vi "dfd_Create Filter Bank Response Distortion.vi"(7 "# freq bins (512)":i32=512, 8 "error in (no error)":errorcluster, 10 "synthesis subband filtes":T1[](array[typedef]) {"mMRate_SumWl" min=1 max=32 step=1; "mMRate_InputIwl" min=1 max=32 step=1; "mMRate_GainWl" min=1 max=32 step=1; "mMRate_OutputWl" min=1 max=32 step=1; "mMRate_InputWl" min=1 max=32 step=1; "mMRate_CoefWl" min=1 max=32 step=1; "mMRate_Mode" items=["Default"=-1, "No Rate Change"=0, "Interpolation"=1, "Decimation"=2, "Interpolated"=3, "Rational"=4]}, 11 "analysis subband filters":T1[](array[typedef]) {"mMRate_SumWl" min=1 max=32 step=1; "mMRate_InputIwl" min=1 max=32 step=1; "mMRate_GainWl" min=1 max=32 step=1; "mMRate_OutputWl" min=1 max=32 step=1; "mMRate_InputWl" min=1 max=32 step=1; "mMRate_CoefWl" min=1 max=32 step=1; "mMRate_Mode" items=["Default"=-1, "No Rate Change"=0, "Interpolation"=1, "Decimation"=2, "Interpolated"=3, "Rational"=4]}) -> (0 "error out":errorcluster, 3 "overall":cdb[](array[numeric]))   [LabVIEW 2017, in "NI_DigFilter_FilterBank.lvlib"]
uses:
  <vilib>/addons/Digital Filter Design/NI_DigFilter_FilterBank.lvlib
  <vilib>/addons/Digital Filter Design/_Objects.llb/DFD Multirate Filter Obj.ctl
  <vilib>/addons/Digital Filter Design/_Objects.llb/DFD Multirate Mode.ctl
  <vilib>/addons/Digital Filter Design/_Objects.llb/DFD Coef Norm Type.ctl
  <vilib>/addons/Digital Filter Design/_Objects.llb/DFD Round-off Mode.ctl
  <vilib>/addons/Digital Filter Design/_Objects.llb/DFD FXP MRate Multiply Mode.ctl
  <vilib>/addons/Digital Filter Design/NI_DigFilterLicensed.lvlib
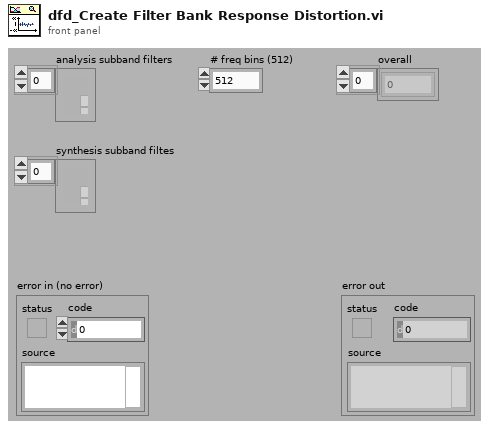
[diagram p1: front panel]
types:
  T1 = typedef "NI_DigFilterLicensed.lvlib/DFD Multirate Filter Obj.ctl" = cluster{"mMRate_Structure":enum16{"CIC", "FIR", "IIR", "Lattice"}, "mMRate_Mode":T2, "mMRate_Factor":i32, "mMRate_FIRParams":cluster{"mMRate_FIR_H":dbl[], "mMRate_FIR_IsNyquist?":bool, "mMRate_FIR_IsSymmetric?":bool}, "mMRate_CICParams":cluster{"mMRate_CIC_#Stage":i32, "mMRate_CIC_Lag":i32, "mMRate_CIC_Type":enum16{"Lowpass", "Highpass"}}, "mMRate_Order":i32, "mMRate_Version":string, "mMRate_Comments":string, "mMRate_RationalFactor":cluster{"mMRate_L":i32, "mMRate_M":i32}, "mMRate_Fs":dbl, "mMRate_Quantized?":bool, "mMRate_QFilterGain":dbl, "mMRate_CoefWl":i16, "mMRate_Scaling":cluster{"mMRate_ScaleByPowerOf2?":bool, "mMRate_ScaleType":T3}, "mMRate_InputWl":i16, "mMRate_OutputWl":i16, "mMRate_OutputMode":T4, "mMRate_MultMode":T5, "mMRate_BitPruning":bool, "mMRate_GainWl":i16, "mMRate_OutputFwl":i16, "mMRate_SumIwl":i16, "mMRate_InputIwl ":i16, "mMRate_SumWl":i16, "mMRate_CoefIwl":i16}
  T2 = typedef "NI_DigFilterLicensed.lvlib/DFD Multirate Mode.ctl" = i16
  T3 = typedef "NI_DigFilterLicensed.lvlib/DFD Coef Norm Type.ctl" = enum16{"No Norm", "Time Domain 1-Norm", "Time Domain 2-Norm", "Time Domain Inf-Norm"}
  T4 = typedef "NI_DigFilterLicensed.lvlib/DFD Round-off Mode.ctl" = enum16{"Nearest", "Truncation"}
  T5 = typedef "NI_DigFilterLicensed.lvlib/DFD FXP MRate Multiply Mode.ctl" = enum16{"Truncated", "Full"}
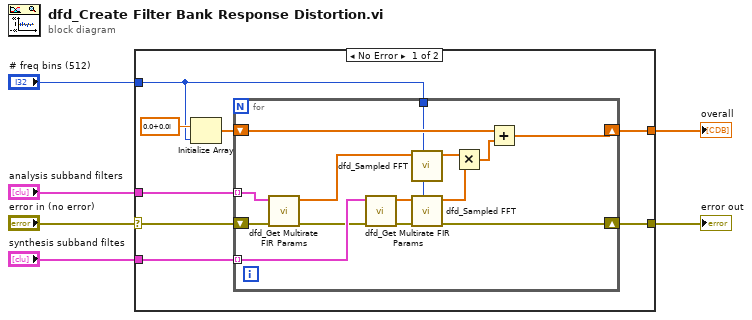
[diagram p0: block diagram]
diagram:
  n1 = case shown="No Error" "error in (no error)" {
    selector: "error in (no error)" -> [w11 w28]
    tunnel: [w9 _] -> w6
    tunnel: "synthesis subband filtes" -> [w7 _]
    tunnel: "analysis subband filters" -> [w8 _]
    tunnel: "# freq bins (512)" -> [w12 _]
    tunnel: [w10 w28] -> w1
    frame No Error {
      n2 = Initialize Array(cdb 0.0+0.0i ("element"), w12) -> (w13:cdb[])
      n3 = for {
        tunnel: w8 -> [w27] mode=indexing
        tunnel: w7 -> [w26] mode=indexing
        tunnel: w12 -> [w18]
        shift-right: [w17] -> w9
        shift-left: w13 -> [w24]
        shift-right: [w19] -> w10
        shift-left: w11 -> [w20]
        n4 = call <vilib>:"dfd_Get Multirate FIR Params.vi"("error in (no error)"=w20, "multirate filter in"=w27) -> ("error out"=w23:errorcluster, "h (n)"=w21:dbl[])  [unwired: 5 in, 3 out]
        n5 = call <vilib>:"dfd_Get Multirate FIR Params.vi"("error in (no error)"=w23, "multirate filter in"=w26) -> ("error out"=w19:errorcluster, "h (n)"=w22:dbl[])  [unwired: 5 in, 3 out]
        n6 = call <vilib>:"dfd_Sampled FFT.vi"("# freq bins (512)"=w18, "h[n]"=w21) -> ("FFT {X}"=w16:cdb[])  [unwired: 9 in]
        n7 = call <vilib>:"dfd_Sampled FFT.vi"("# freq bins (512)"=w18, "h[n]"=w22) -> ("FFT {X}"=w25:cdb[])  [unwired: 9 in]
        n8 = Multiply(x=w16, y=w25) -> (x*y=w15:cdb[])
        n9 = Add(x=w24, y=w15) -> (x+y=w17:cdb[])
      }
    }
    frame Error {
    }
  }
  "overall" <- w6
  "error out" <- w1
